vi "Update Timestamp.vi"(8 "error in (no error)":errorcluster, 11 "Packet in":refnum<class "Packet.lvclass">) -> (0 "error out":errorcluster, 3 "Packet out":refnum<class "Packet.lvclass">)   [LabVIEW 2020, in "Communication Classes.lvlib" / "Packet.lvclass"]
uses:
  Packet.lvclass
  Packet.lvclass/Packet.ctl
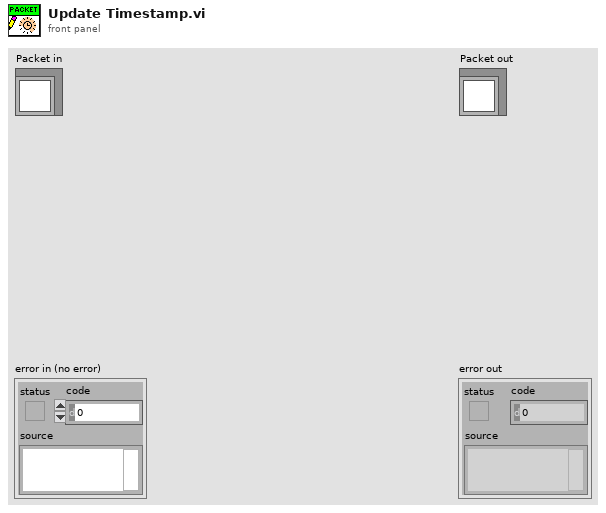
[diagram p1: front panel]
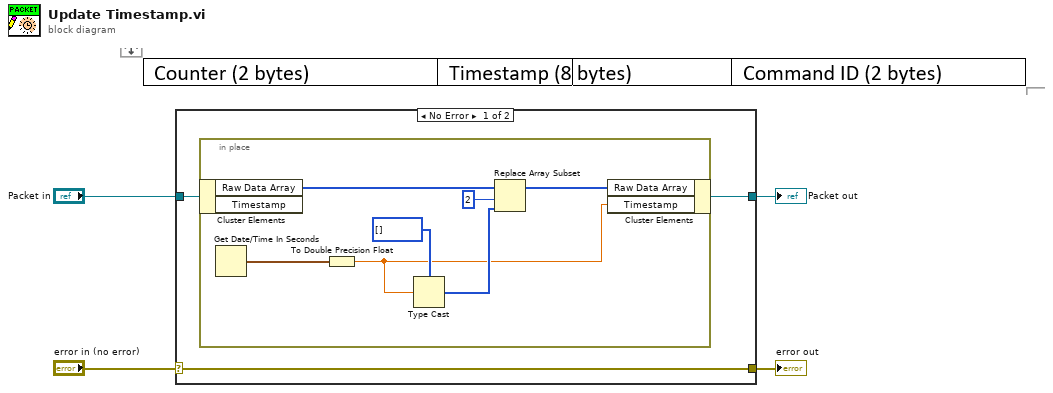
[diagram p0: block diagram]
diagram:
  n1 = case shown="No Error" "error in (no error)" {
    selector: "error in (no error)" -> [w7 w15]
    tunnel: [w7 w15] -> w3
    tunnel: [w5 w16] -> w1
    tunnel: "Packet in" -> [w6 w16]
    frame No Error {
      n2 = in-place {
        n3 = in-place-cluster #1(w6) -> ("Raw Data Array"=w14:u8[])  [unwired: 1 out]
        n4 = Get Date/Time In Seconds() -> (seconds since 1Jan1904=w11:timestamp)
        n5 = To Double Precision Float(number=w11) -> (double precision float=w8:dbl)
        n6 = Type Cast(type=u8[] [], x=w8) -> (*(type *) &x=w9:u8[])
        n7 = Replace Array Subset "Replace Array Subset"(array=w14, new element=w9, index=2) -> (w13:u8[])
        n8 = in-place-cluster #1("Raw Data Array"=w13, "Timestamp"=w8) -> (w5:refnum<class "Packet.lvclass">)
      }
    }
    frame Error {
    }
  }
  "error out" <- w3
  "Packet out" <- w1
